vi "Control Offset.vi"() -> (3 "Offset From Tab Edge in (px)":i32=5)   [LabVIEW 2014]
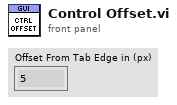
[diagram p1: front panel]
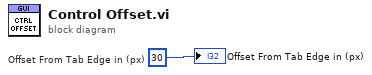
[diagram p0: block diagram]
diagram:
  w1 = 30  # Offset From Tab Edge in (px)
  "Offset From Tab Edge in (px)" <- w1
